vi "average-4.21.vi"(1 "Numeric 2":dbl, 2 "Numeric":dbl) -> (0 "Numeric 3":dbl)   [LabVIEW 2015]
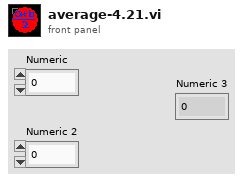
[diagram p1: front panel]
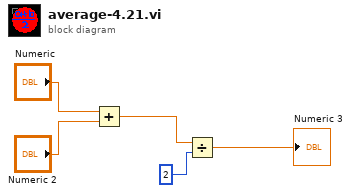
[diagram p0: block diagram]
diagram:
  n1 = Add(x="Numeric", y="Numeric 2") -> (x+y=w3:dbl)
  n2 = Divide(x=w3, y=2) -> (x/y=→"Numeric 3":dbl)
